vi "Edit Connector Pane Multiple.vi"(11 "error in (no error)":errorcluster) -> (15 "error out":errorcluster)   [LabVIEW 2021, in "Migrator.lvlib"]
uses:
  Migrator.lvlib
  Migrator Reusables/Migrator Reusables.lvlib
  Path Functions/Path Functions.lvlib
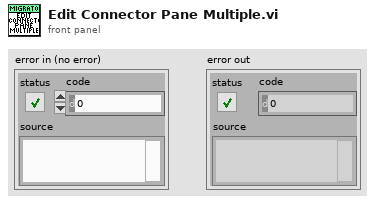
[diagram p1: front panel]
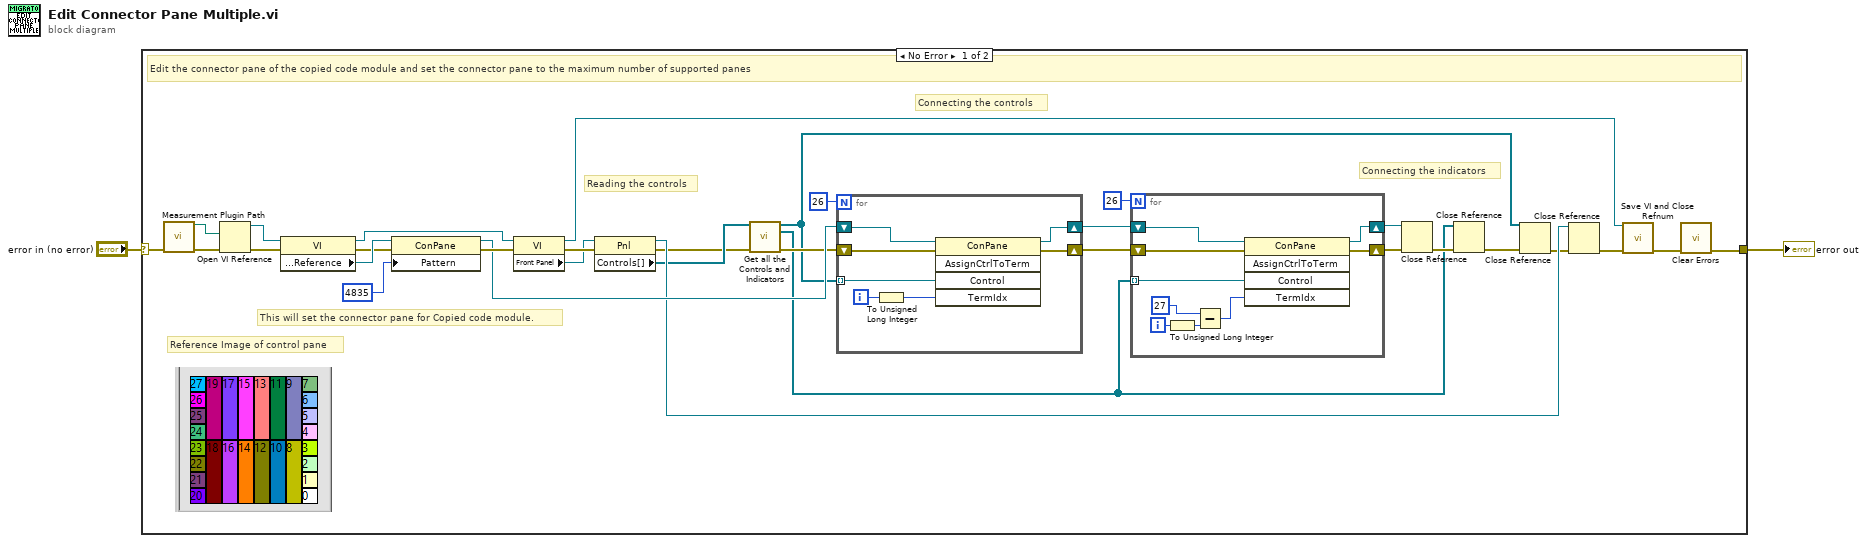
[diagram p0: block diagram]
diagram:
  n1 = case shown="No Error" "error in (no error)" {
    selector: "error in (no error)" -> [w5 w51]
    tunnel: [w6 w51] -> w1
    frame No Error {
      # "Reference Image of control pane"
      # "Connecting the indicators"
      # "Connecting the controls"
      # "Reading the controls"
      # "This will set the connector pane for Copied code module."
      # "Edit the connector pane of the copied code module and set the connector pane to the maximum number of supported panes"
      n2 = call "Measurement Plugin Path.vi"("error in (no error)"=w5) -> ("New Code Module"=w3:path, "error out"=w4:errorcluster)  [unwired: 2 in, 11 out]
      n3 = Open VI Reference(vi path=w3, error in (no error)=w4) -> (vi reference=w23:refnum<vi>, error out=w29:errorcluster)  [unwired: 1 in, 3 out]
      n4 = property class="VI"(reference=w23, error in=w29) -> (reference out=w34:refnum<vi>, error out=w30:errorcluster, "Connector Pane:Reference"=w32:refnum<vi>)
      n5 = property class="ConPane"(reference=w32, error in=w30, "Pattern"=u32 4835) -> (reference out=w28:refnum<vi>, error out=w31:errorcluster)
      n6 = property class="VI"(reference=w34, error in=w31) -> (reference out=w19:refnum<vi>, error out=w33:errorcluster, "Front Panel"=w20:refnum<vi>)
      n7 = property class="Pnl"(reference=w20, error in=w33) -> (reference out=w18:refnum<vi>, error out=w7:errorcluster, "Controls[]"=w8:refnum<vi>[])
      n8 = call "Get all the Controls and Indicators.vi"("Controls[]"=w8, "error in (no error)"=w7) -> ("Controls[]"=w13:refnum<vi>[], "Indicators[]"=w9:refnum<vi>[], "error out"=w16:errorcluster)  [unwired: 11 in]
      n9 = for {
        N: 26 -> [_]
        tunnel: w13 -> [w38] mode=indexing
        shift-right: [w37] -> w25
        shift-left: w16 -> [w40]
        shift-right: [w39] -> w27
        shift-left: w28 -> [w41]
        i -> [w36]
        n10 = To Unsigned Long Integer(number=w36) -> (unsigned 32bit integer=w35:u32)
        n11 = invoke class="ConPane" method="AssignCtrlToTerm"(reference=w41, error in=w40, "Control"=w38, "TermIdx"=w35) -> (reference out=w39:refnum<vi>, error out=w37:errorcluster)  [unwired: 1 in, 3 out]
      }
      n12 = for {
        N: 26 -> [_]
        tunnel: w9 -> [w47] mode=indexing
        shift-right: [w46] -> w24
        shift-left: w25 -> [w49]
        shift-right: [w48] -> w26
        shift-left: w27 -> [w50]
        i -> [w45]
        n13 = To Unsigned Long Integer(number=w45) -> (unsigned 32bit integer=w42:u32)
        n14 = Subtract(x=u32 27 ("Terminal Index"), y=w42) -> (x-y=w43:u32)
        n15 = invoke class="ConPane" method="AssignCtrlToTerm"(reference=w50, error in=w49, "Control"=w47, "TermIdx"=w43) -> (reference out=w48:refnum<vi>, error out=w46:errorcluster)  [unwired: 1 in, 3 out]
      }
      n16 = Close Reference(reference=w26, error in (no error)=w24) -> (error out=w10:errorcluster)
      n17 = Close Reference(reference=w9, error in (no error)=w10) -> (error out=w11:errorcluster)
      n18 = Close Reference(reference=w13, error in (no error)=w11) -> (error out=w12:errorcluster)
      n19 = Close Reference(reference=w18, error in (no error)=w12) -> (error out=w17:errorcluster)
      n20 = call "Save VI and Close Refnum.vi"("VI Refnum"=w19, "error in"=w17) -> ("error out"=w21:errorcluster)  [unwired: 13 in]
      n21 = call <vilib>:"Clear Errors.vi"("error in (no error)"=w21) -> ("error out"=w6:errorcluster)  [unwired: 5 in, 1 out]
    }
    frame Error {
    }
  }
  "error out" <- w1
